vi "DOE Dryer PreCondition Build States.vi"(8 "Error In":errorcluster, 9 "Step 3":bool, 10 "Step 2":bool, 11 "Step 1":bool) -> (0 "Error Out":errorcluster, 3 "States Out":string)   [LabVIEW 2016]
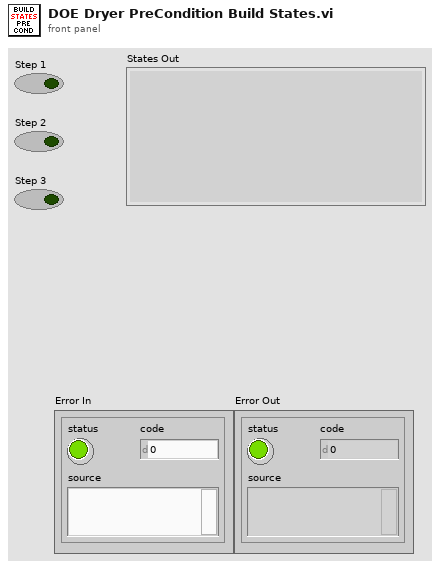
[diagram p1: front panel]
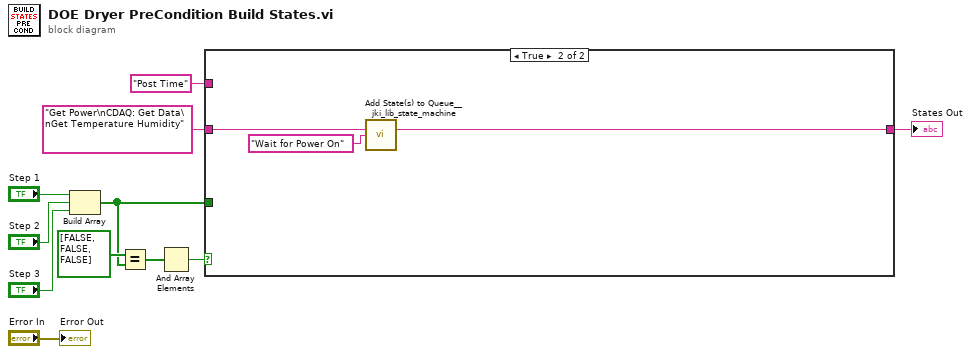
[diagram p0: block diagram]
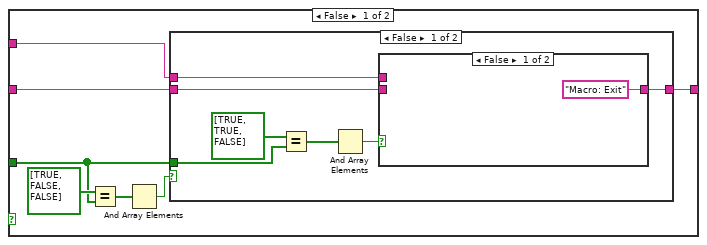
[diagram p2: hidden frame]
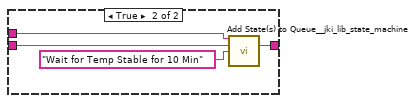
[diagram p3: hidden frame]
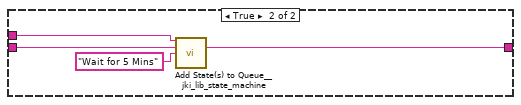
[diagram p4: hidden frame]
diagram:
  n1 = Build Array("Step 1", "Step 2", "Step 3") -> (w2:bool[])
  n2 = Equal?(x=bool[] [FALSE, FALSE, FALSE], y=w2) -> (x = y?=w6:bool[])
  n3 = And Array Elements(Boolean array=w6) -> (logical AND=w5:bool)
  n4 = case shown="True" w5 {
    tunnel: "Post Time" ("State(s) in Front (\"\")") -> [w16 _]
    tunnel: "Get Power\nCDAQ: Get Data\nGet Temperature Humidity" ("State(s) in Front (\"\")") -> [w15 w37]
    tunnel: [w14 w35] -> w1
    tunnel: w2 -> [w12 _]
    frame False {
      n5 = Equal?(x=bool[] [TRUE, FALSE, FALSE], y=w12) -> (x = y?=w18:bool[])
      n6 = And Array Elements(Boolean array=w18) -> (logical AND=w13:bool)
      n7 = case shown="False" w13 {
        tunnel: w16 -> [w21 w33]
        tunnel: w15 -> [w20 w32]
        tunnel: [w19 w31] -> w14
        tunnel: w12 -> [w23 _]
        frame False {
          n8 = Equal?(x=bool[] [TRUE, TRUE, FALSE], y=w23) -> (x = y?=w24:bool[])
          n9 = And Array Elements(Boolean array=w24) -> (logical AND=w22:bool)
          n10 = case shown="False" w22 {
            tunnel: w21 -> [_ w30]
            tunnel: w20 -> [_ w29]
            tunnel: ["Macro: Exit" ("States Out") w27] -> w19
            frame False {
            }
            frame True {
              n11 = call <vilib>:"Add State(s) to Queue__jki_lib_state_machine.vi"("State(s) in Front (\"\")"=w30, "State(s) in (\"\")"=w29, "State(s) at Back (\"\")"="Wait for Temp Stable for 10 Min" ("State(s) in Front (\"\")")) -> ("States Out"=w27:string)  [unwired: 12 in]
            }
          }
        }
        frame True {
          n12 = call <vilib>:"Add State(s) to Queue__jki_lib_state_machine.vi"("State(s) in Front (\"\")"=w33, "State(s) in (\"\")"=w32, "State(s) at Back (\"\")"="Wait for 5 Mins" ("State(s) in Front (\"\")")) -> ("States Out"=w31:string)  [unwired: 12 in]
        }
      }
    }
    frame True {
      n13 = call <vilib>:"Add State(s) to Queue__jki_lib_state_machine.vi"("State(s) in (\"\")"=w37, "State(s) at Back (\"\")"="Wait for Power On" ("State(s) in Front (\"\")")) -> ("States Out"=w35:string)  [unwired: 13 in]
    }
  }
  "States Out" <- w1
  "Error Out" <- "Error In"
